vi "minimum detection.vi"(7 "Sens":dbl, 9 "Vnoise":dbl, 10 "Pelletron Volts":dbl, 11 "Velocity":dbl) -> (3 "Minimum Detection":dbl)   [LabVIEW 2012]
panel:
  out "output variable":dbl
  out "Vnoise/sense":dbl
  # "Minimum detection=2*vnoise/sens*pelletronvolts./v.^2;"
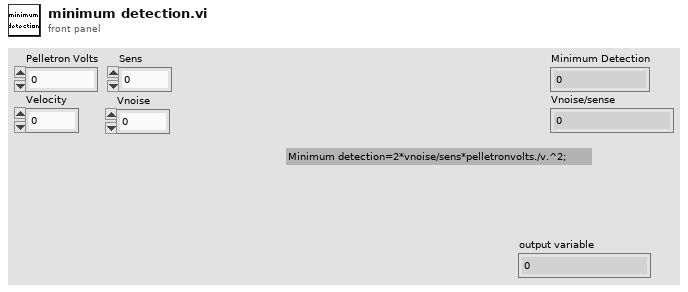
[diagram p1: front panel]
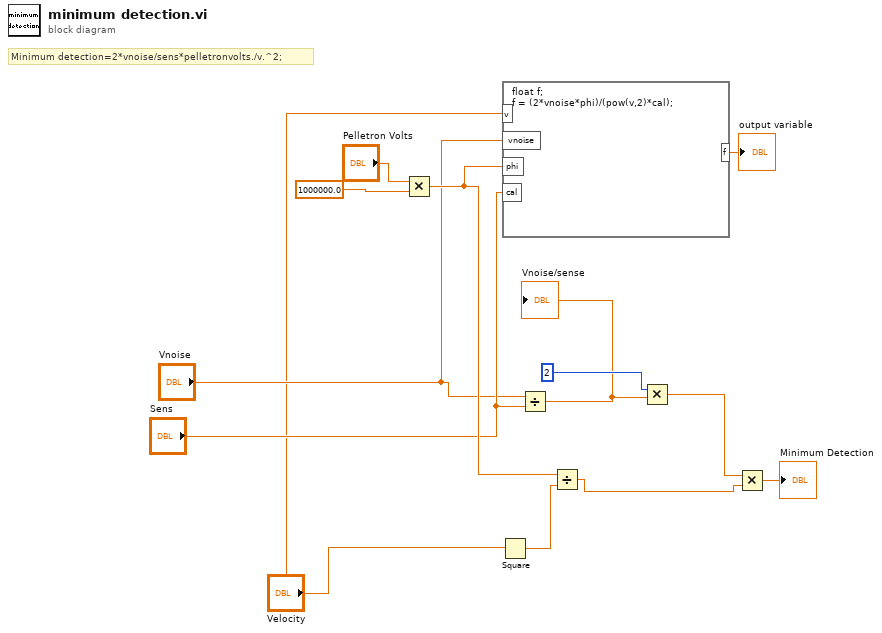
[diagram p0: block diagram]
diagram:
  # "Minimum detection=2*vnoise/sens*pelletronvolts./v.^2;"
  n1 = Multiply(x="Pelletron Volts", y=1000000.0) -> (x*y=w5:dbl)
  n2 = Square(x="Velocity") -> (x^2=w12:dbl)
  n3 = formula code="float f;\nf = (2*vnoise*phi)/(pow(v,2)*cal);"("v"="Velocity", "vnoise"="Vnoise", "phi"=w5, "cal"="Sens") -> ("f"=→"output variable":dbl)
  n4 = Divide(x="Vnoise", y="Sens") -> (x/y=w9:dbl)
  "Vnoise/sense" <- w9
  n5 = Divide(x=w5, y=w12) -> (x/y=w11:dbl)
  n6 = Multiply(x=2, y=w9) -> (x*y=w8:dbl)
  n7 = Multiply(x=w8, y=w11) -> (x*y=→"Minimum Detection":dbl)
